vi "PXI-AO Queue.vi"() -> (8 "Queue":refnum<queue>)   [LabVIEW 2020]
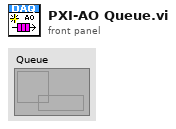
[diagram p1: front panel]
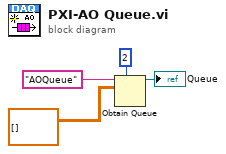
[diagram p0: block diagram]
diagram:
  n1 = Obtain Queue(max queue size (-1, unlimited)=2, name (unnamed)="AOQueue", element data type=dbl[][] []) -> (queue out=→"Queue":refnum<queue>)  [unwired: 2 in, 2 out]
